vi "Lock-in Digital Port Control.vi"(8 "error in (no error)":errorcluster, 11 "Hardware Parameters":T1={"Scan Calibration [G/V]"=0.0, "Modulation Calibration [G/V]"=0.0, "Modulation Phase [deg]"=0.0, "Modulation Frequency [Hz]"=0.0, "Attenuation [dB]"=0, "Input Channel Count"=0, "Time constant"=7, "Sensitivity"=17, "Frequency Output Voltage [V]"=0.0, "Phase Output Voltage [V]"=0.0, "Lock-in Offset Compensation"=FALSE, "RF [GHz]"=0.0, "Q Start"=0.0, "Q End"=0.0, "Balance"=0.0, "Phase Error"=0.0, "AFC Error"=0.0, "AFC"=FALSE, "Magnet Rotation"=FALSE, "Balance Scaling Factor"=1.0, "Phase Error Scaling Factor"=1.0, "AFC Error Scaling Factor"=1.0, "Frequency Counter ID"="", "Sweep Waveform"=enum."Sawtooth", "Q-Factor Scale"=0.0, " Q-Data Scale"=0.0, " Q-Data Offset"=0.0, "Magnet Rotation Slope"=0.0, "Magnet Rotation Offset"=0.0, "Phase Sweep Resolution"=0.0, "Hardware Version Number"="", "Spectrometer ID Number"=0, "Spectrometer Name"="", "Lock in Saturation"=0.0, "Balance Threshold"=0.0, "Phase Error Threshold"=0.0, "AFC Error Threshold"=0.0, "Linear Actuator Length"=0.0, "Lock-in OK?"=FALSE, "Ignore Lock-in Comm. Failure"=FALSE, "Gradient Addresses"=[], "Gradient Calibrations [G/A*mm]"=[], "Gradient Power Supplies"=[], "Lock-in Address"="", "Magnet Type"=enum."RRI", "Camera Names"=[], "Sweep Limit [Gauss]"=0.0, "Modulation Limit [Gauss]"=0.0, "Balance Threshold Exceeded?"=FALSE, "Phase Threshold Exceeded?"=FALSE, "AFC Threshold Exceeded?"=FALSE, "Consecutive Re-tune attempts"=0, "Reverse Sweep Slope [sec]"=0.0, "Reverse Sweep Offset [G]"=0.0, "AFC Field Correction [V/MHz]"=0.0, "Active Gradients (X Y Z)"=[], "SpO2 Calibration [SpO2/V]"=1.0, "Heart Rate Calibration [BPM/V]"=1.0, "Thermocouple Channel"=""} {"Sensitivity" items=["", "2 nV", "5 nV", "10 nV", "20 nV", "50 nV", "100 nV", "200 nV", "500 nV", "1 uV", "2 uV", "5 uV", "10 uV", "20 uV", "50 uV", "100 uV", "200 uV", "500 uV", "1 mV", "2 mV", "5 mV", "10 mV", "20 mV", "50 mV", "100 mV", "200 mV", "500 mV", "1 V"]; "Time constant" items=["10 us", "20 us", "40 us", "80 us", "160 us", "320 us", "640 us", "5 ms", "10 ms", "20 ms", "50 ms", "100 ms", "200 ms", "500 ms", "1 s", "2 s", "5 s", "10 s", "20 s", "50 s", "100 s", "200 s", "500 s", "1 ks", "2 ks", "5 ks", "10 ks", "20 ks", "50 ks", "100 ks"]}) -> (0 "error out":errorcluster)   [LabVIEW 2016]
uses:
  Types/Hardware Parameters.ctl
  <vilib>/Instr/_visa.llb/VISA Open Access Mode.ctl
panel:
  # "Bridge I/O"
  # "Magnet Rotation"
  # "Field Calibration"
  # "Lock In Amplifier"
  # "Spectrometer Information"
  # "DAQ Settings"
  # "Gradient Coils and Field"
  # "X"
  # "Y"
  # "Z"
  # "Q-Measurements"
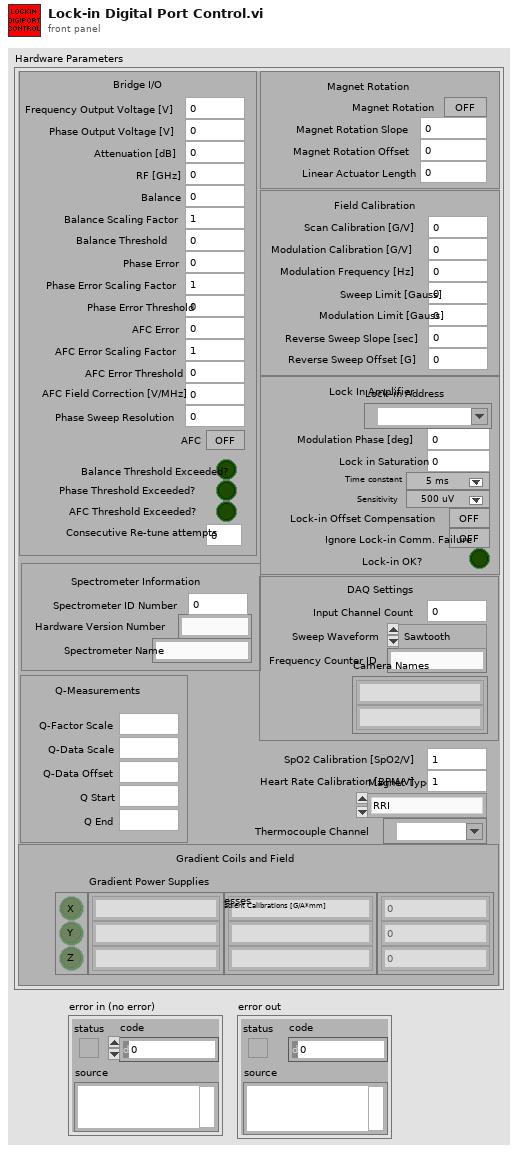
[diagram p1: front panel]
types:
  T1 = typedef "Hardware Parameters.ctl" = cluster{"Scan Calibration [G/V]":dbl, "Modulation Calibration [G/V]":dbl, "Modulation Phase [deg]":dbl, "Modulation Frequency [Hz]":dbl, "Attenuation [dB]":u16, "Input Channel Count":i32, "Time constant":u16, "Sensitivity":u16, "Frequency Output Voltage [V]":dbl, "Phase Output Voltage [V]":dbl, "Lock-in Offset Compensation":bool, "RF [GHz]":dbl, "Q Start":dbl, "Q End":dbl, "Balance":dbl, "Phase Error":dbl, "AFC Error":dbl, "AFC":bool, "Magnet Rotation":bool, "Balance Scaling Factor":dbl, "Phase Error Scaling Factor":dbl, "AFC Error Scaling Factor":dbl, "Frequency Counter ID":string, "Sweep Waveform":enum16{"Sine Wave", "Square Wave", "Sawtooth", "Triangle Wave"}, "Q-Factor Scale":dbl, " Q-Data Scale":dbl, " Q-Data Offset":dbl, "Magnet Rotation Slope":dbl, "Magnet Rotation Offset":dbl, "Phase Sweep Resolution":dbl, "Hardware Version Number":string, "Spectrometer ID Number":i32, "Spectrometer Name":string, "Lock in Saturation":dbl, "Balance Threshold":dbl, "Phase Error Threshold":dbl, "AFC Error Threshold":dbl, "Linear Actuator Length":dbl, "Lock-in OK?":bool, "Ignore Lock-in Comm. Failure":bool, "Gradient Addresses":string[], "Gradient Calibrations [G/A*mm]":dbl[], "Gradient Power Supplies":string[], "Lock-in Address":refnum<visa-resource-name>, "Magnet Type":enum16{"RRI", "BARDA", "Whole Body Permanent", "RRI Electromagnet"}, "Camera Names":string[], "Sweep Limit [Gauss]":dbl, "Modulation Limit [Gauss]":dbl, "Balance Threshold Exceeded?":bool, "Phase Threshold Exceeded?":bool, "AFC Threshold Exceeded?":bool, "Consecutive Re-tune attempts":i32, "Reverse Sweep Slope [sec]":dbl, "Reverse Sweep Offset [G]":dbl, "AFC Field Correction [V/MHz]":dbl, "Active Gradients (X Y Z)":bool[], "SpO2 Calibration [SpO2/V]":dbl, "Heart Rate Calibration [BPM/V]":dbl, "Thermocouple Channel":tag}
  T2 = typedef "VISA Open Access Mode.ctl" = u32
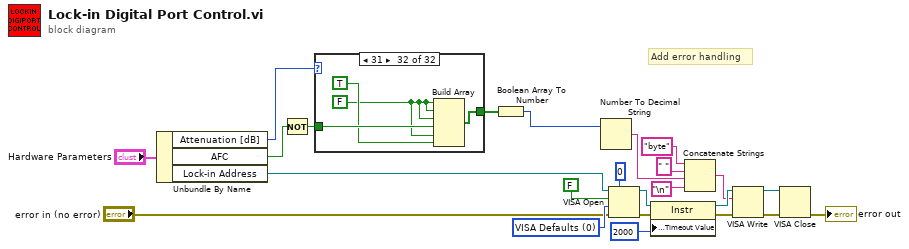
[diagram p0: block diagram]
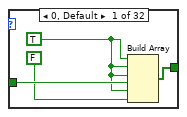
[diagram p2: hidden frame]
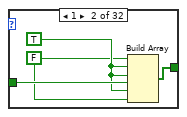
[diagram p3: hidden frame]
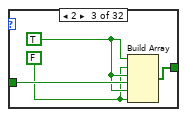
[diagram p4: hidden frame]
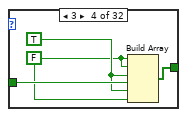
[diagram p5: hidden frame]
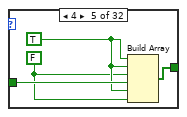
[diagram p6: hidden frame]
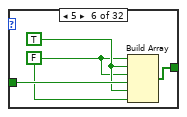
[diagram p7: hidden frame]
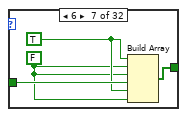
[diagram p8: hidden frame]
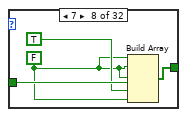
[diagram p9: hidden frame]
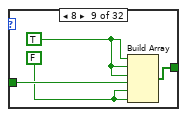
[diagram p10: hidden frame]
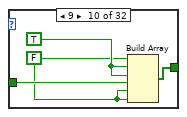
[diagram p11: hidden frame]
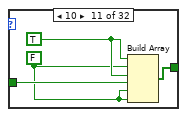
[diagram p12: hidden frame]
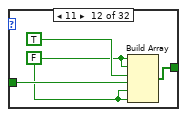
[diagram p13: hidden frame]
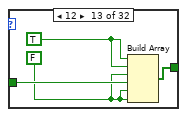
[diagram p14: hidden frame]
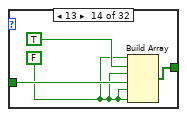
[diagram p15: hidden frame]
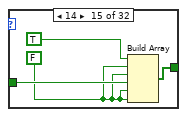
[diagram p16: hidden frame]
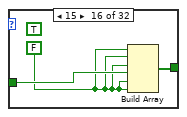
[diagram p17: hidden frame]
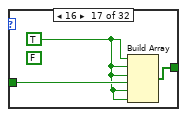
[diagram p18: hidden frame]
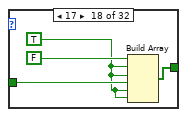
[diagram p19: hidden frame]
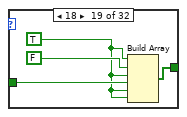
[diagram p20: hidden frame]
diagram:
  w24 = T2 0 items=["VISA Defaults"=0, "Exclusive Lock"=1, "Load Configured Settings"=4] ("Access Mode")
  # "Add error handling"
  n1 = Unbundle By Name("Hardware Parameters") -> ("Attenuation [dB]"=w1:u16, "AFC"=w2:bool, "Lock-in Address"=w3:refnum<visa-resource-name>)
  n2 = Not(x=w2) -> (.not. x?=w6:bool)
  n3 = case shown="31" w1 {
    tunnel: w6 -> [w28 w32 w36 w40 w44 w48 w52 w56 w60 w64 w68 w72 w76 w80 w84 w87 w90 w94 w98 w102 w106 w110 w114 w118 w122 w126 w130 w134 w138 w142 w146 w150]
    tunnel: [w27 w31 w35 w39 w43 w47 w51 w55 w59 w63 w67 w71 w75 w79 w83 w86 w89 w93 w97 w101 w105 w109 w113 w117 w121 w125 w129 w133 w137 w141 w145 w149] -> w7
    frame 0, Default {
      w25 = TRUE
      n4 = Build Array(w25, w25, w25, w28, w25, FALSE) -> (w27:bool[])
    }
    frame 1 {
      w30 = TRUE
      w29 = FALSE
      n5 = Build Array(w29, w30, w30, w32, w30, w29) -> (w31:bool[])
    }
    frame 2 {
      w34 = TRUE
      w33 = FALSE
      n6 = Build Array(w34, w33, w34, w36, w34, w33) -> (w35:bool[])
    }
    frame 3 {
      w38 = TRUE
      w37 = FALSE
      n7 = Build Array(w37, w37, w38, w40, w38, w37) -> (w39:bool[])
    }
    frame 4 {
      w42 = TRUE
      w41 = FALSE
      n8 = Build Array(w42, w42, w41, w44, w42, w41) -> (w43:bool[])
    }
    frame 5 {
      w46 = TRUE
      w45 = FALSE
      n9 = Build Array(w45, w46, w45, w48, w46, w45) -> (w47:bool[])
    }
    frame 6 {
      w50 = TRUE
      w49 = FALSE
      n10 = Build Array(w50, w49, w49, w52, w50, w49) -> (w51:bool[])
    }
    frame 7 {
      w53 = FALSE
      n11 = Build Array(w53, w53, w53, w56, TRUE, w53) -> (w55:bool[])
    }
    frame 8 {
      w58 = TRUE
      w57 = FALSE
      n12 = Build Array(w58, w58, w58, w60, w57, w57) -> (w59:bool[])
    }
    frame 9 {
      w62 = TRUE
      w61 = FALSE
      n13 = Build Array(w61, w62, w62, w64, w61, w61) -> (w63:bool[])
    }
    frame 10 {
      w66 = TRUE
      w65 = FALSE
      n14 = Build Array(w66, w65, w66, w68, w65, w65) -> (w67:bool[])
    }
    frame 11 {
      w69 = FALSE
      n15 = Build Array(w69, w69, TRUE, w72, w69, w69) -> (w71:bool[])
    }
    frame 12 {
      w74 = TRUE
      w73 = FALSE
      n16 = Build Array(w74, w74, w73, w76, w73, w73) -> (w75:bool[])
    }
    frame 13 {
      w77 = FALSE
      n17 = Build Array(w77, TRUE, w77, w80, w77, w77) -> (w79:bool[])
    }
    frame 14 {
      w81 = FALSE
      n18 = Build Array(TRUE, w81, w81, w84, w81, w81) -> (w83:bool[])
    }
    frame 15 {
      (unwired) TRUE
      w85 = FALSE
      n19 = Build Array(w85, w85, w85, w87, w85, w85) -> (w86:bool[])
    }
    frame 16 {
      w88 = TRUE
      (unwired) FALSE
      n20 = Build Array(w88, w88, w88, w90, w88, w88) -> (w89:bool[])
    }
    frame 17 {
      w91 = TRUE
      n21 = Build Array(FALSE, w91, w91, w94, w91, w91) -> (w93:bool[])
    }
    frame 18 {
      w95 = TRUE
      n22 = Build Array(w95, FALSE, w95, w98, w95, w95) -> (w97:bool[])
    }
    frame 19 {
      w99 = TRUE
      w100 = FALSE
      n23 = Build Array(w100, w100, w99, w102, w99, w99) -> (w101:bool[])
    }
    frame 20 {
      w104 = TRUE
      n24 = Build Array(w104, w104, FALSE, w106, w104, w104) -> (w105:bool[])
    }
    frame 21 {
      w108 = TRUE
      w107 = FALSE
      n25 = Build Array(w107, w108, w107, w110, w108, w108) -> (w109:bool[])
    }
    frame 22 {
      w112 = TRUE
      w111 = FALSE
      n26 = Build Array(w112, w111, w111, w114, w112, w112) -> (w113:bool[])
    }
    frame 23 {
      w116 = TRUE
      w115 = FALSE
      n27 = Build Array(w115, w115, w115, w118, w116, w116) -> (w117:bool[])
    }
    frame 24 {
      w119 = TRUE
      n28 = Build Array(w119, w119, w119, w122, FALSE, w119) -> (w121:bool[])
    }
    frame 25 {
      w124 = TRUE
      w123 = FALSE
      n29 = Build Array(w123, w124, w124, w126, w123, w124) -> (w125:bool[])
    }
    frame 26 {
      w128 = TRUE
      w127 = FALSE
      n30 = Build Array(w128, w127, w128, w130, w127, w128) -> (w129:bool[])
    }
    frame 27 {
      w132 = TRUE
      w131 = FALSE
      n31 = Build Array(w131, w131, w132, w134, w131, w132) -> (w133:bool[])
    }
    frame 28 {
      w136 = TRUE
      w135 = FALSE
      n32 = Build Array(w136, w136, w135, w138, w135, w136) -> (w137:bool[])
    }
    frame 29 {
      w140 = TRUE
      w139 = FALSE
      n33 = Build Array(w139, w140, w139, w142, w139, w140) -> (w141:bool[])
    }
    frame 30 {
      w144 = TRUE
      w143 = FALSE
      n34 = Build Array(w144, w143, w143, w146, w143, w144) -> (w145:bool[])
    }
    frame 31 {
      w147 = FALSE
      n35 = Build Array(w147, w147, w147, w150, w147, TRUE) -> (w149:bool[])
    }
  }
  n36 = Boolean Array To Number(Boolean array=w7) -> (number=w5:u32)
  n37 = Number To Decimal String(number=w5) -> (decimal integer string=w8:string)  [unwired: 1 in]
  n38 = VISA Open(timeout (0)=u32 0 ("General Settings:Timeout Value"), duplicate session (F)=FALSE, access mode=w24, error in (no error)="error in (no error)", VISA resource name=w3) -> (VISA resource name=w22:refnum<visa-resource-name>, error out=w21:errorcluster)
  n39 = property class="Instr"(reference=w22, error in=w21, "General Settings:Timeout Value"=u32 2000) -> (reference out=w20:refnum<visa-resource-name>, error out=w19:errorcluster)
  n40 = Concatenate Strings("byte" ("string"), " " ("string"), w8, "\n") -> (w16:string)
  n41 = VISA Write(VISA resource name=w20, write buffer=w16, error in (no error)=w19) -> (VISA resource name out=w12:refnum<visa-resource-name>, error out=w13:errorcluster)  [unwired: 1 out]
  n42 = VISA Close(VISA resource name=w12, error in (no error)=w13) -> (error out=→"error out":errorcluster)
